vi "Command_Drive_Time.vi"(0 "Startup":bool, 1 "Speed_X":dbl, 2 "Speed_Y":dbl, 3 "Timeout":dbl=3.0) -> (5 "Reinit":bool, 6 "Completed":bool=TRUE, 7 "Speeds":dbl[](array[numeric]))   [LabVIEW 2018]
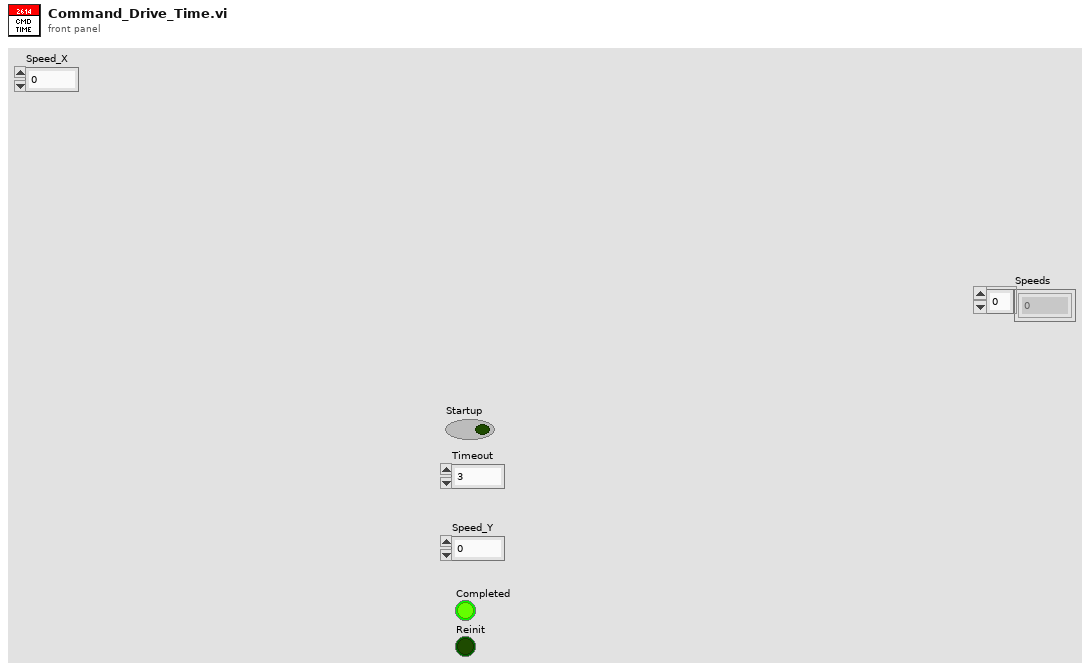
[diagram p1: front panel]
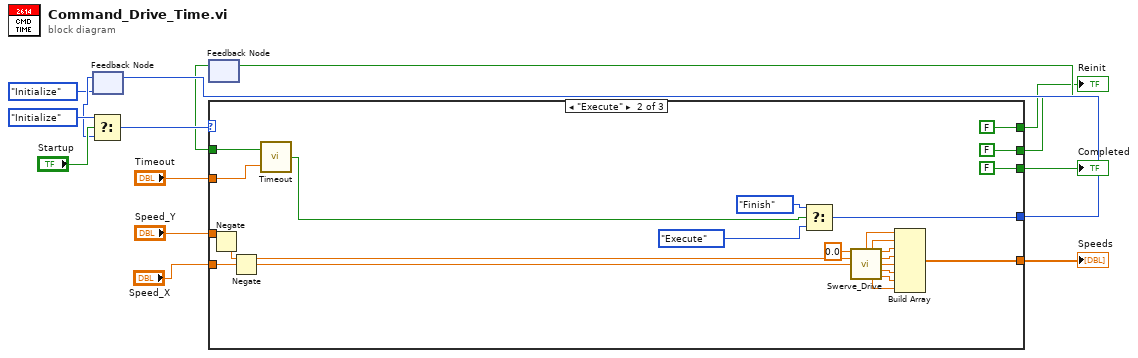
[diagram p0: block diagram]
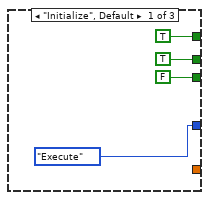
[diagram p2: hidden frame]
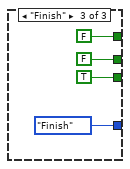
[diagram p3: hidden frame]
diagram:
  n1 = feedback #1(enum16{"Initialize", "Execute", "Finish"}."Initialize" ("f")) -> (w10:enum16{"Initialize", "Execute", "Finish"})
  n2 = Select(t=enum16{"Initialize", "Execute", "Finish"}."Initialize", s="Startup", f=w10) -> (s? t:f=w14:enum16{"Initialize", "Execute", "Finish"})
  n3 = feedback #2() -> (w8:bool)  [unwired: 1 in]
  n4 = case shown="\"Execute\"" w14 {
    tunnel: [enum16{"Initialize", "Execute", "Finish"}."Execute" w38 enum16{"Initialize", "Execute", "Finish"}."Finish" ("f")] -> w11
    tunnel: w8 -> [_ w36 _]
    tunnel: [TRUE FALSE FALSE] -> w9
    tunnel: [FALSE FALSE TRUE] -> w7
    tunnel: [TRUE FALSE FALSE] -> w6
    tunnel: "Timeout" -> [_ w34 _]
    tunnel: "Speed_Y" -> [_ w23 _]
    tunnel: [_ w25 _] -> w2
    tunnel: "Speed_X" -> [_ w22 _]
    frame "Initialize", Default {
    }
    frame "Execute" {
      n5 = Negate(x=w23) -> (-x=w20:dbl)
      n6 = Negate(x=w22) -> (-x=w19:dbl)
      n7 = call "Timeout.vi"("Timeout"=w34, "Initialize"=w36) -> ("Timed Out?"=w24:bool)
      n8 = Select(t=enum16{"Initialize", "Execute", "Finish"}."Finish", s=w24, f=enum16{"Initialize", "Execute", "Finish"}."Execute") -> (s? t:f=w38:enum16{"Initialize", "Execute", "Finish"})
      n9 = call "Swerve_Drive.vi"("Z"=0.0, "Y"=w20, "X"=w19) -> ("Back Left Spin Speed"=w33:dbl, "Back Right Spin Speed"=w32:dbl, "Front Left Spin Speed"=w31:dbl, "Front Right Spin Speed"=w30:dbl, "Back Left Motor Power"=w29:dbl, "Back Right Motor Power"=w28:dbl, "Front Right Motor Power"=w26:dbl, "Front Left Motor Power"=w27:dbl)  [unwired: 5 in]
      n10 = Build Array(w33, w32, w31, w30, w29, w28, w27, w26) -> (w25:dbl[])
    }
    frame "Finish" {
    }
  }
  "Completed" <- w7
  "Reinit" <- w6
  "Speeds" <- w2
  n11 = feedback-in #1(w11) -> ()
  n12 = feedback-in #2(w9) -> ()
